vi "SVT Human Vibration Weighting Filter (Fixed Rates) (N Ch).vi"(6 "reset filter (F)":bool, 8 "error in (no error)":errorcluster, 10 "weighting":u16(ring) items=["Linear"=0, "Wh: hand-arm"=13, "Wb: vertical whole-body"=8, "Wc: horizontal whole-body"=9, "Wd: horizontal whole-body"=10, "We: rotational whole-body"=11, "Wj: vertical head"=14, "Wk: vertical whole-body"=15, "Wm: whole-body in buildings"=16, "Wf: low-frequency whole-body"=12], 11 "scaled signals [EU]":waveform(dbl)[](array[waveform])) -> (0 "error out":errorcluster, 3 "weighted signals [EU]":waveform(dbl)[](array[waveform]))   [LabVIEW 2017, in "SoundVib_HumanVibration.lvlib"]
doc: "Applies the selected human vibration weighting to a scaled signal expressed in engineering units. This VI complies with ISO 8041:2005 (E), JIS B 7760:2004, and JISB 7761:2004 standards. Each instance of this VI maintains its own state; use the N Channel instance of this VI to process an array of channels. This VI operates on time-continuous data; it resets on a discontinuity. Wire data to the <B>scaled signal [EU]</B> input to determine the polymorphic instance to use or manually select the instance."
uses:
  <vilib>/addons/Sound and Vibration/svt_Weighting/SoundVib_HumanVibration.lvlib
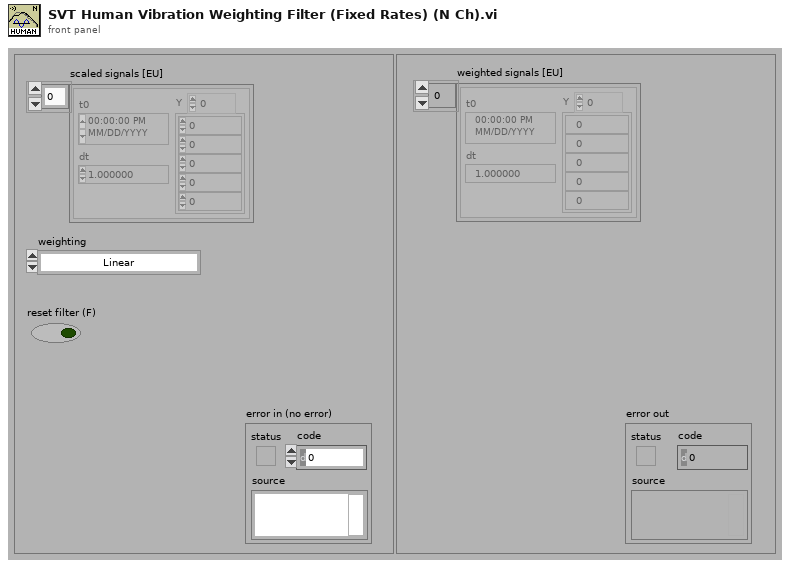
[diagram p1: front panel]
types:
  T1 = typedef "svc_Weighting Filter Text Ring.ctl" = u16
  T2 = cluster{"filter structure":enum32{"IIR 2nd Order", "IIR 4th Order"}, "Reverse Coefficients":dbl[], "Forward Coefficients":dbl[]}
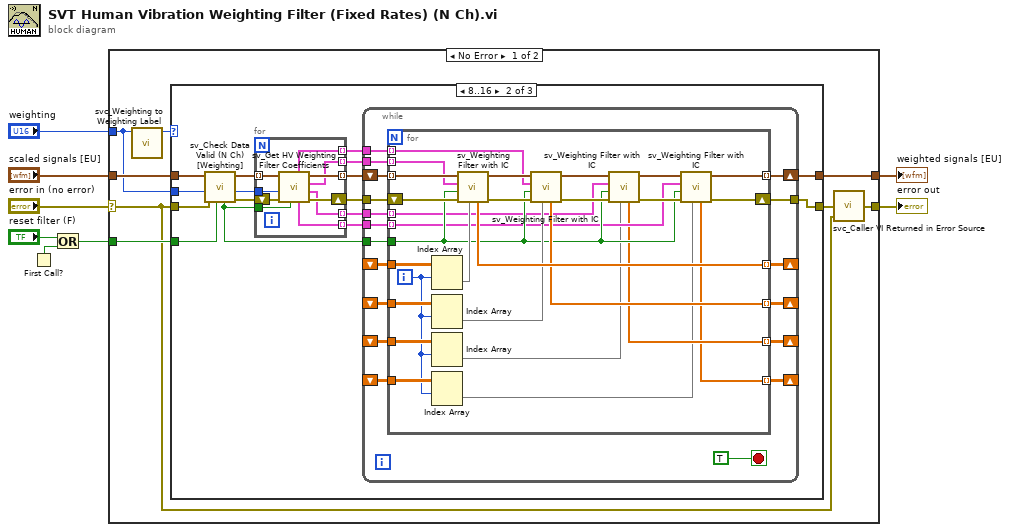
[diagram p0: block diagram]
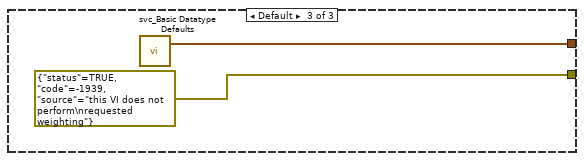
[diagram p3: hidden frame]
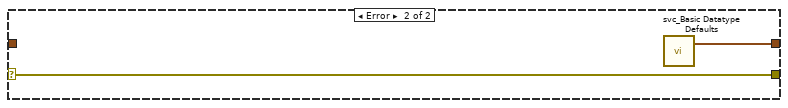
[diagram p4: hidden frame]
diagram:
  n1 = First Call?() -> (First Call?: T/F=w7:bool)
  n2 = Or(x="reset filter (F)", y=w7) -> (x .or. y?=w3:bool)
  n3 = case shown="No Error" "error in (no error)" {
    selector: "error in (no error)" -> [w9 w94]
    tunnel: "scaled signals [EU]" -> [w16 _]
    tunnel: [w12 w94] -> w5
    tunnel: [w14 w93] -> w4
    tunnel: w3 -> [w13 _]
    tunnel: "weighting" -> [w11 _]
    frame No Error {
      n4 = call <vilib>:"svc_Weighting to Weighting Label.vi"("weighting filter"=w11) -> ("weighting enum"=w10:T1)  [unwired: 9 in, 1 out]
      n5 = case shown="8..16" w10 {
        tunnel: w9 -> [w17 w30 _]
        tunnel: w16 -> [w18 w34 _]
        tunnel: [w17 w33 errorcluster {"status"=TRUE, "code"=-1939, "source"="this VI does not perform\nrequested weighting"} ("error out")] -> w15
        tunnel: [w18 w32 w92] -> w14
        tunnel: w13 -> [_ w31 _]
        tunnel: w11 -> [_ w29 _]
        frame 0 {
        }
        frame 8..16 {
          n6 = call <vilib>:"sv_Check Data Valid (N Ch) [Weighting].vi"("reset (in)"=w31, "error in (no error)"=w30, "weighting"=w29, "scaled signal [in]"=w34) -> ("error out"=w26:errorcluster, "weighting"=w23:T1, "scaled signal [out]"=w27:waveform(dbl)[], "reset (out)"=w22:bool)  [unwired: 4 in]
          n7 = for {
            tunnel: w27 -> [w44] mode=indexing
            tunnel: w23 -> [w39]
            tunnel: [w42] -> w24 mode=indexing
            tunnel: [w40] -> w28 mode=indexing
            tunnel: w22 -> [w38]
            shift-right: [w41] -> w25
            shift-left: w26 -> [w43]
            tunnel: [w37] -> w21 mode=indexing
            tunnel: [w36] -> w20 mode=indexing
            tunnel: [w35] -> w19 mode=indexing
            n8 = call <vilib>:"sv_Get HV Weighting Filter Coefficients.vi"("reset filter (F)"=w38, "error in (no error)"=w43, "weighting filter"=w39, "scaled signal"=w44) -> ("error out"=w41:errorcluster, "a-v filter coefficients"=w36:T2, "LP filter coefficients"=w40:T2, "dup scaled signal"=w42:waveform(dbl), "upward step filter coefficients"=w35:T2, "HP filter coefficients"=w37:T2)  [unwired: 2 in]
          }
          n9 = while {
            tunnel: w22 -> [w59]
            tunnel: [w54] -> w33
            shift-left: _ -> [w55]
            shift-right: [w62] -> _
            tunnel: w25 -> [w56]
            tunnel: w28 -> [w57]
            shift-right: [w60] -> w32
            shift-left: w24 -> [w58]
            shift-right: [w52] -> _
            shift-left: _ -> [w53]
            tunnel: w21 -> [w51]
            tunnel: w20 -> [w50]
            tunnel: w19 -> [w49]
            shift-right: [w48] -> _
            shift-left: _ -> [w47]
            shift-right: [w45] -> _
            shift-left: _ -> [w46]
            stop <- TRUE stop-if-true
            n10 = for {
              tunnel: w55 -> [w90]
              tunnel: [w89] -> w62 mode=indexing
              tunnel: w58 -> [w88] mode=indexing
              tunnel: w57 -> [w64] mode=indexing
              tunnel: [w79] -> w60 mode=indexing
              tunnel: w59 -> [w74]
              shift-right: [w78] -> w54
              shift-left: w56 -> [w87]
              tunnel: w53 -> [w77]
              tunnel: [w76] -> w52 mode=indexing
              tunnel: w51 -> [w63] mode=indexing
              tunnel: w50 -> [w73] mode=indexing
              tunnel: w49 -> [w72] mode=indexing
              tunnel: w47 -> [w71]
              tunnel: [w70] -> w48 mode=indexing
              tunnel: w46 -> [w68]
              tunnel: [w65] -> w45 mode=indexing
              i -> [w67]
              n11 = Index Array(array=w90, index (row)=w67) -> (element=w86:dbl[])  [unwired: 1 in]
              n12 = Index Array(array=w77, index (row)=w67) -> (element=w75:dbl[])  [unwired: 1 in]
              n13 = Index Array(array=w71, index (row)=w67) -> (element=w69:dbl[])  [unwired: 1 in]
              n14 = Index Array(array=w68, index (row)=w67) -> (element=w66:dbl[])  [unwired: 1 in]
              n15 = call <vilib>:"sv_Weighting Filter with IC.vi"("Initial Filter State"=w86, "error in (no error)"=w87, "reset filter (F)"=w74, "filter coefficients"=w64, "signal [V]"=w88) -> ("error out"=w82:errorcluster, "filtered signal [EU]"=w83:waveform(dbl), "Final Filter State"=w89:dbl[])  [unwired: 4 in]
              n16 = call <vilib>:"sv_Weighting Filter with IC.vi"("Initial Filter State"=w75, "error in (no error)"=w82, "reset filter (F)"=w74, "filter coefficients"=w63, "signal [V]"=w83) -> ("error out"=w85:errorcluster, "filtered signal [EU]"=w84:waveform(dbl), "Final Filter State"=w76:dbl[])  [unwired: 4 in]
              n17 = call <vilib>:"sv_Weighting Filter with IC.vi"("Initial Filter State"=w69, "error in (no error)"=w85, "reset filter (F)"=w74, "filter coefficients"=w73, "signal [V]"=w84) -> ("error out"=w81:errorcluster, "filtered signal [EU]"=w80:waveform(dbl), "Final Filter State"=w70:dbl[])  [unwired: 4 in]
              n18 = call <vilib>:"sv_Weighting Filter with IC.vi"("Initial Filter State"=w66, "error in (no error)"=w81, "reset filter (F)"=w74, "filter coefficients"=w72, "signal [V]"=w80) -> ("error out"=w78:errorcluster, "filtered signal [EU]"=w79:waveform(dbl), "Final Filter State"=w65:dbl[])  [unwired: 4 in]
            }
          }
        }
        frame Default {
          n19 = call <vilib>:"svc_Basic Datatype Defaults.vi"() -> ("empty array of waveforms"=w92:waveform(dbl)[])  [unwired: 7 in, 12 out]
        }
      }
      n20 = call <vilib>:"svc_Caller VI Returned in Error Source.vi"("warning input to caller"=w9, "error in (no error)"=w15) -> ("error out"=w12:errorcluster)  [unwired: 3 in]
    }
    frame Error {
      n21 = call <vilib>:"svc_Basic Datatype Defaults.vi"() -> ("empty array of waveforms"=w93:waveform(dbl)[])  [unwired: 7 in, 12 out]
    }
  }
  "weighted signals [EU]" <- w4
  "error out" <- w5
